vi "Connection successful.vi"(8 "error in":errorcluster, 10 "Connected?":bool, 11 "Module ID":i32=-1) -> (0 "error out":errorcluster)   [LabVIEW 2020, in "Arduino-Adafruit stepper.lvlib"]
doc: "Broadcasts when a successful connection has been established with the Arduino.\n_____\nCreated using DQMH Event Scripter 7.0.1.1316."
uses:
  Arduino-Adafruit stepper.lvlib
  Connection successful Argument--cluster.ctl
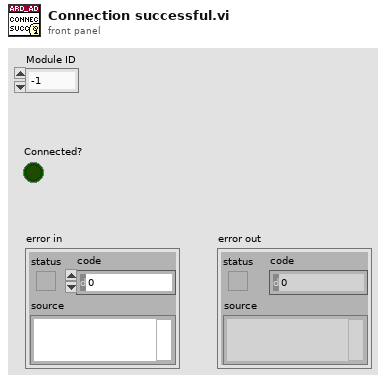
[diagram p1: front panel]
types:
  T1 = typedef "Arduino-Adafruit stepper.lvlib/Connection successful Argument--cluster.ctl" = cluster{"Module ID":i32, "Connected?":bool}
  T2 = typedef "Arduino-Adafruit stepper.lvlib/Broadcast Events--cluster.ctl" = cluster{"Module Did Init":refnum<user-event>, "Status Updated":refnum<user-event>, "Error Reported":refnum<user-event>, "Module Did Stop":refnum<user-event>, "Update Module Execution Status":refnum<user-event>, "Connection successful":refnum<user-event>, "Connection failed":refnum<user-event>, "Device disconnected":refnum<user-event>, "Motors ready":refnum<user-event>, "System busy":refnum<user-event>, "State info available":refnum<user-event>, "Home reached":refnum<user-event>, "End position reached":refnum<user-event>}
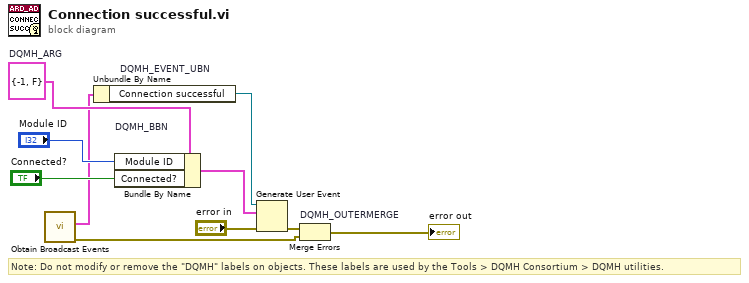
[diagram p0: block diagram]
diagram:
  w5 = T1 {"Module ID"=-1, "Connected?"=FALSE}  # DQMH_ARG
  # "Note: Do not modify or remove the \"DQMH\" labels on objects. These labels are used by the Tools > DQMH Consortium > DQMH utilities."
  n1 = call "Obtain Broadcast Events.vi"() -> ("error out"=w2:errorcluster, "Arduino-Adafruit stepper Broadcast Events"=w1:T2)  [unwired: 10 in]
  n2 = Unbundle By Name "DQMH_EVENT_UBN"(w1) -> ("Connection successful"=w7:refnum<user-event>)
  n3 = Bundle By Name "DQMH_BBN"(cluster=w5, "Module ID"="Module ID", "Connected?"="Connected?") -> (w8:T1)
  n4 = Generate User Event(user event=w7, event data cluster=w8, error in="error in") -> (error out=w6:errorcluster)  [unwired: 1 in, 1 out]
  n5 = Merge Errors "DQMH_OUTERMERGE"(w6, w2) -> (→"error out":errorcluster)
